vi "Get Installed Projects.vi"(8 "Error In":errorcluster, 11 "Sync Source Config":T1) -> (0 "Error Out":errorcluster, 2 "Installed Projects":string[](array[string]), 3 "Sync Source Config":T1)   [LabVIEW 2011, in "LVH-Build-Tools.lvlib"]
doc: "Get all installed projects and the LV versions each project is installed to."
uses:
  <vilib>/LabVIEW Hacker/Build Tools/LVH-Build-Tools.lvlib
  Type Defs/Sync Source Configuration.ctl
  Type Defs/Installed Project.ctl
  Local Toolbox/_Installed LabVIEW Version.ctl
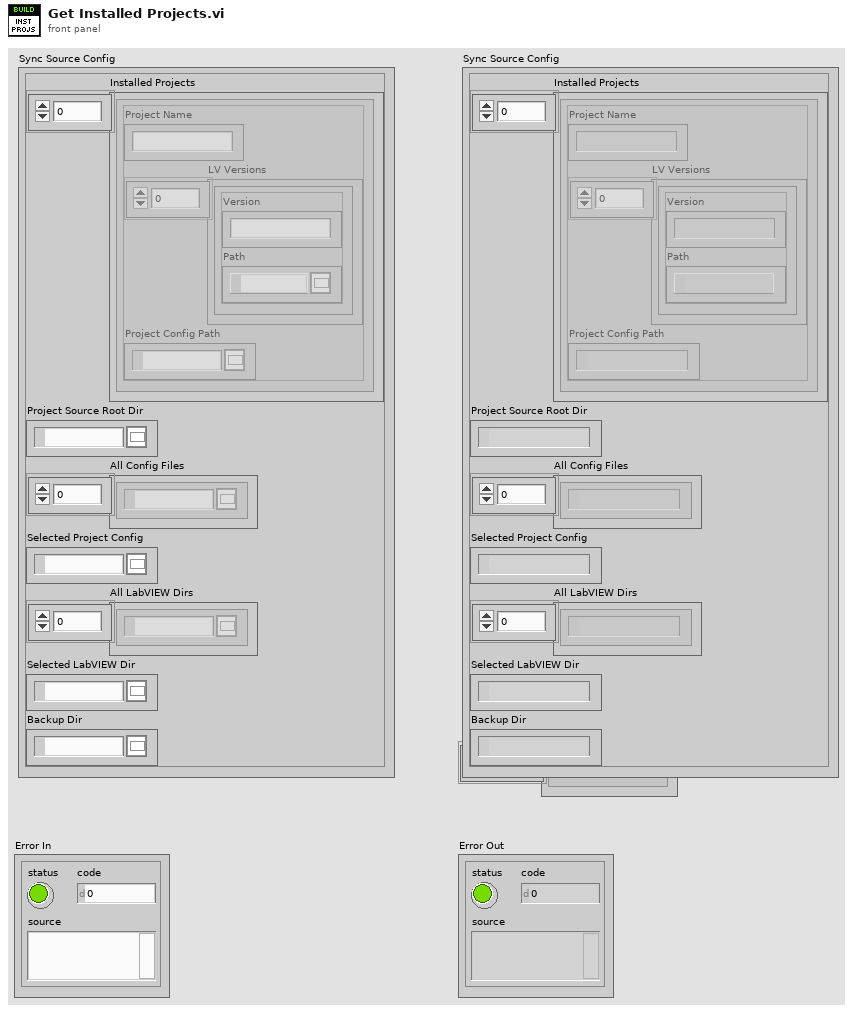
[diagram p1: front panel]
types:
  T1 = typedef "LVH-Build-Tools.lvlib/Sync Source Configuration.ctl" = cluster{"Installed Projects":T2[], "Project Source Root Dir":path, "All Config Files":path[], "Selected Project Config":path, "All LabVIEW Dirs":path[], "Selected LabVIEW Dir":path, "Backup Dir":path}
  T2 = typedef "LVH-Build-Tools.lvlib/Installed Project.ctl" = cluster{"Project Name":string, "LV Versions":T3[], "Project Config Path":path}
  T3 = typedef "LVH-Build-Tools.lvlib/_Installed LabVIEW Version.ctl" = cluster{"Version":string, "Path":path}
  T4 = typedef "LVH-Build-Tools.lvlib/Configuration.ctl" = cluster{"Source Root":path, "Install Root":string, "Components":string[], "Ignore":string[], "Config Files":path[], "LV Directories":path[], "Install Paths":T5}
  T5 = typedef "LVH-Build-Tools.lvlib/Install Configuration.ctl" = cluster{"LabVIEW Directory":path, "Project Source Config":path}
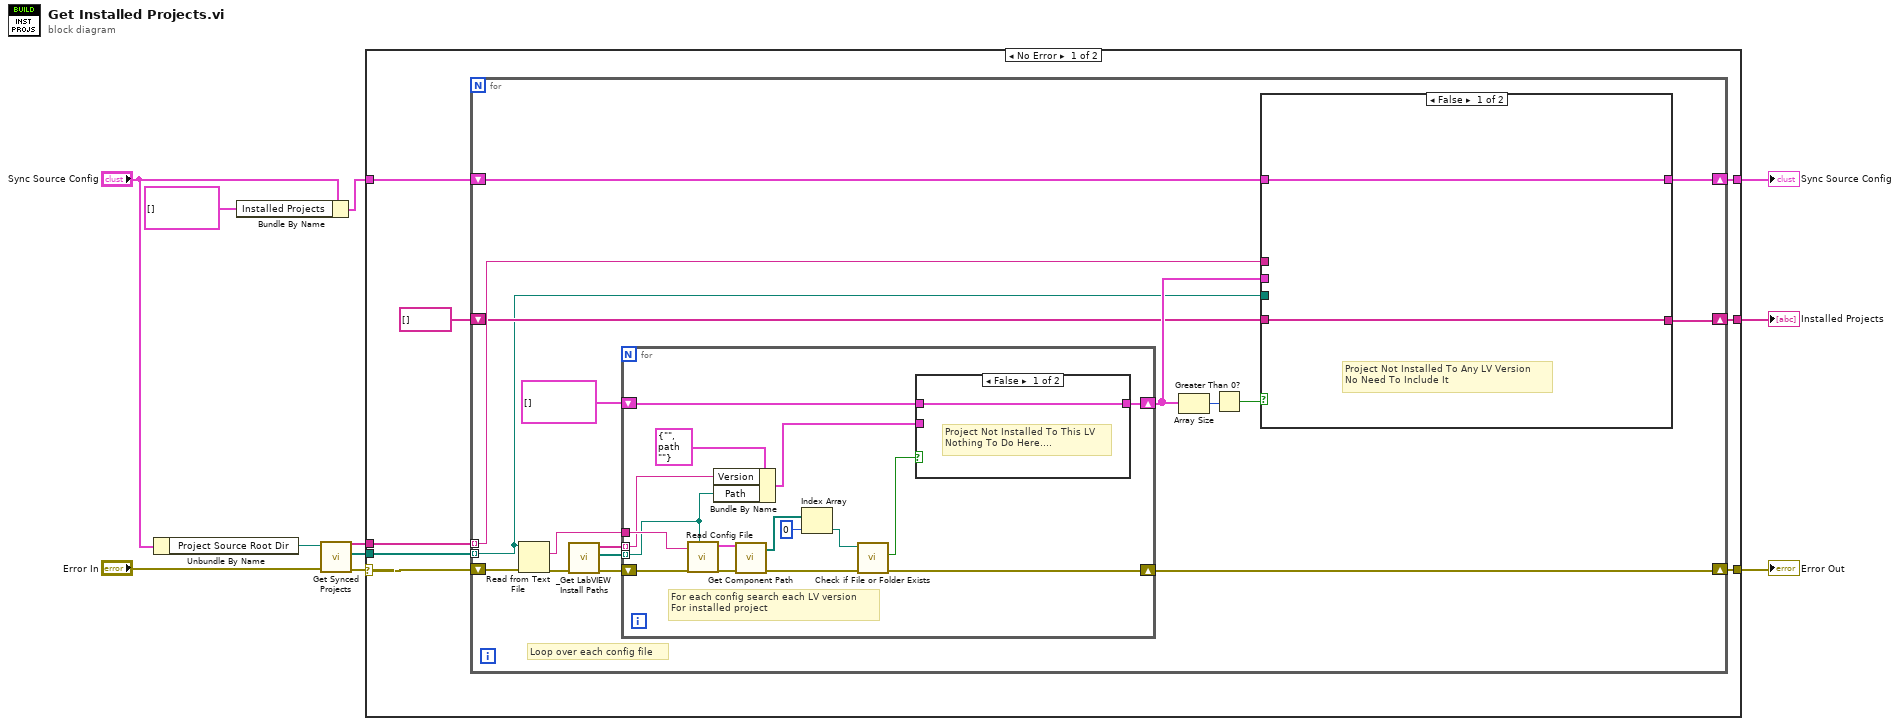
[diagram p0: block diagram]
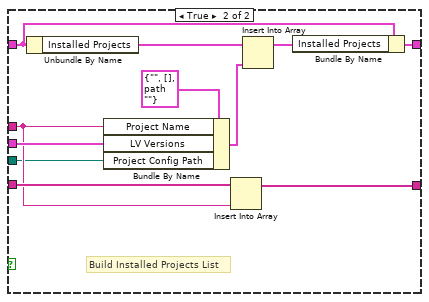
[diagram p2: hidden frame]
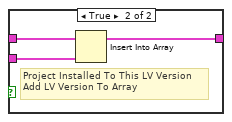
[diagram p3: hidden frame]
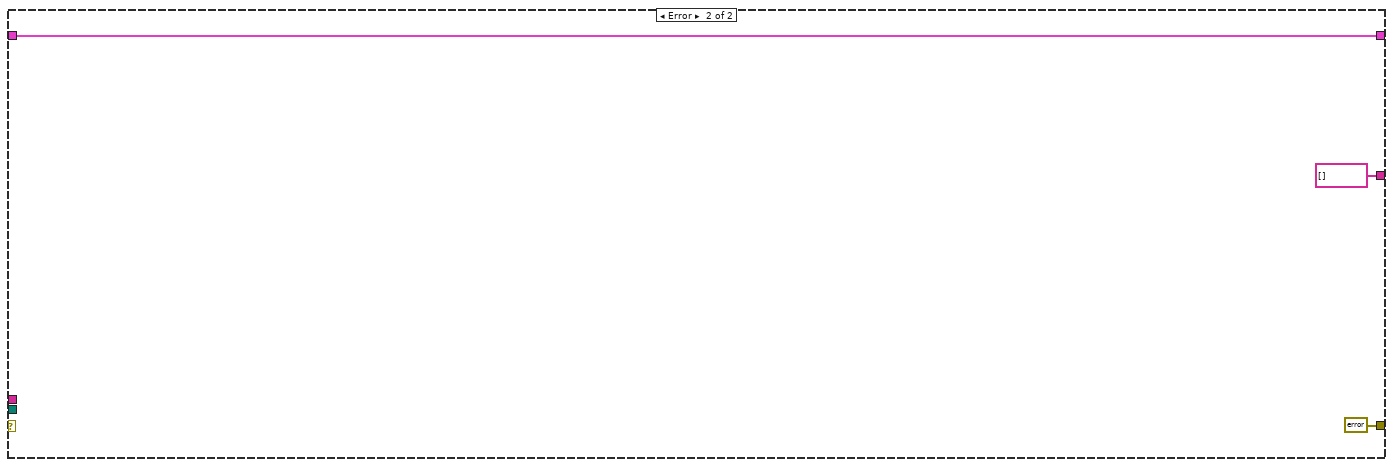
[diagram p4: hidden frame]
diagram:
  n1 = Unbundle By Name("Sync Source Config") -> ("Project Source Root Dir"=w5:path)
  n2 = Bundle By Name(cluster="Sync Source Config", "Installed Projects"=T2[] []) -> (w1:T1)
  n3 = call "Get Synced Projects.vi"("Error In"="Error In", "Source Root"=w5) -> ("Error Out"=w4:errorcluster, "Config File Paths"=w8:path[], "Synced Projects"=w9:string[])  [unwired: 7 in]
  n4 = case shown="No Error" w4 {
    selector: w4 -> [w12 _]
    tunnel: [w19 errorcluster {"status"=FALSE, "code"=0, "source"=""} ("error IO")] -> w11
    tunnel: [w18 w72] -> w10
    tunnel: w9 -> [w17 _]
    tunnel: w8 -> [w16 _]
    tunnel: [w14 string[] []] -> w6
    tunnel: w1 -> [w13 w72]
    frame No Error {
      n5 = for {
        tunnel: w16 -> [w20] mode=indexing
        shift-right: [w29] -> w19
        shift-left: w12 -> [w36]
        tunnel: w17 -> [w28] mode=indexing
        shift-right: [w26] -> w18
        shift-left: w13 -> [w27]
        shift-right: [w21] -> w14
        shift-left: string[] [] -> [w22]
        # "Loop over each config file"
        n6 = Read from Text File(file (use dialog)=w20, error in=w36) -> (text=w35:string, error out=w34:errorcluster)  [unwired: 2 in, 2 out]
        n7 = call "_Get LabVIEW Install Paths.vi"("Error In"=w34) -> ("Error Out"=w33:errorcluster, "LV Directories"=w32:path[], "LV Version"=w31:string[])  [unwired: 8 in]
        n8 = for {
          tunnel: w35 -> [w65]
          tunnel: w32 -> [w50] mode=indexing
          tunnel: w31 -> [w52] mode=indexing
          shift-right: [w55] -> w25
          shift-left: T3[] [] -> [w56]
          shift-right: [w54] -> w29
          shift-left: w33 -> [w62]
          # "For each config search each LV version \nFor installed project"
          n9 = call "Read Config File.vi"("LabVIEW Dir Override"=w50, "error in (no error)"=w62, "Config File In"=w65) -> ("error out"=w63:errorcluster, "Configuration out"=w64:T4)  [unwired: 7 in]
          n10 = Bundle By Name(cluster=T3 {"Version"="", "Path"=path ""} ("Installed LV Version"), "Version"=w52, "Path"=w50) -> (w51:T3)
          n11 = call "Get Component Path.vi"("Error In"=w63, "Configuration"=w64) -> ("Error Out"=w58:errorcluster, "Component Install Paths"=w61:path[])  [unwired: 7 in, 1 out]
          n12 = Index Array(array=w61, index=0) -> (element=w59:path)
          n13 = call <vilib>:"Check if File or Folder Exists.vi"("error in (no error)"=w58, "path"=w59) -> ("error out"=w54:errorcluster, "file or folder exists?"=w57:bool)  [unwired: 7 in, 1 out]
          n14 = case shown="False" w57 {
            tunnel: w56 -> [w66 w69]
            tunnel: [w66 w68] -> w55
            tunnel: w51 -> [_ w67]
            frame False {
              # "Project Not Installed To This LV\nNothing To Do Here...."
            }
            frame True {
              # "Project Installed To This LV Version\nAdd LV Version To Array"
              n15 = Insert Into Array(array=w69, new element=w67) -> (w68:T3[])  [unwired: 1 in]
            }
          }
        }
        n16 = Array Size(array=w25) -> (size(s)=w24:i32)
        n17 = Greater Than 0?(x=w24) -> (x > 0?=w23:bool)
        n18 = case shown="False" w23 {
          tunnel: w25 -> [_ w48]
          tunnel: w28 -> [_ w41]
          tunnel: w27 -> [w38 w44]
          tunnel: [w38 w43] -> w26
          tunnel: w22 -> [w37 w42]
          tunnel: [w37 w40] -> w21
          tunnel: w20 -> [_ w39]
          frame False {
            # "Project Not Installed To Any LV Version\nNo Need To Include It"
          }
          frame True {
            # "Build Installed Projects List"
            n19 = Unbundle By Name(w44) -> ("Installed Projects"=w47:T2[])
            n20 = Bundle By Name(cluster=T2 {"Project Name"="", "LV Versions"=[], "Project Config Path"=path ""} ("Installed Project"), "Project Name"=w41, "LV Versions"=w48, "Project Config Path"=w39) -> (w46:T2)
            n21 = Insert Into Array(array=w42, new element=w41) -> (w40:string[])  [unwired: 1 in]
            n22 = Insert Into Array(array=w47, new element=w46) -> (w45:T2[])  [unwired: 1 in]
            n23 = Bundle By Name(cluster=w44, "Installed Projects"=w45) -> (w43:T1)
          }
        }
      }
    }
    frame Error {
    }
  }
  "Error Out" <- w11
  "Installed Projects" <- w6
  "Sync Source Config" <- w10
